vi "Query.vi"(11 "VISA resource name":refnum<visa-resource-name>) -> (0 "error out":errorcluster, 1 "Instrument Firmware Revision":string, 3 "VISA resource name out":refnum<visa-resource-name>)   [LabVIEW 2018, in "Suita SPAW7000.lvlib"]
doc: "Queries the current instrument firmware revision and instrument driver revision.\n\nRefer to the Readme file for detailed driver information including modification history."
uses:
  <instrlib>/Suita SPAW7000/Suita SPAW7000.lvlib
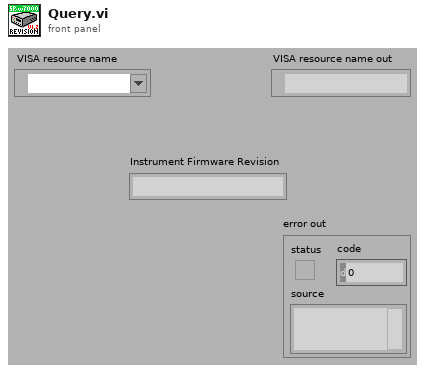
[diagram p1: front panel]
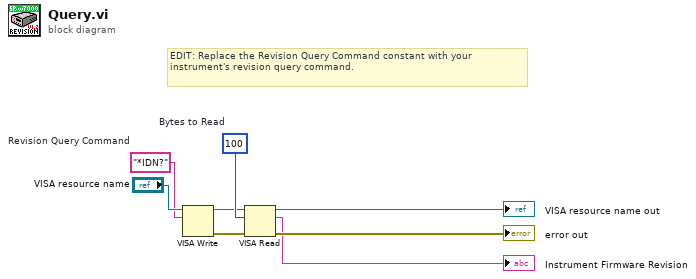
[diagram p0: block diagram]
diagram:
  w4 = "*IDN?"  # Revision Query Command
  w7 = u32 100  # Bytes to Read
  # "EDIT: Replace the Revision Query Command constant with your instrument's revision query command."
  n1 = VISA Write(VISA resource name="VISA resource name", write buffer=w4) -> (VISA resource name out=w6:refnum<visa-resource-name>, error out=w5:errorcluster)  [unwired: 1 in, 1 out]
  n2 = VISA Read(VISA resource name=w6, byte count=w7, error in (no error)=w5) -> (VISA resource name out=→"VISA resource name out":refnum<visa-resource-name>, read buffer=→"Instrument Firmware Revision":string, error out=→"error out":errorcluster)  [unwired: 1 out]
